vi "XLP80_FGlob_CalculatedAnalog.vi"(5 "Function (Recall One)":T2=enum."Recall one", 7 "CalculatedAnalog_Items":T1, 8 "err in":errorcluster caption="error", 10 "Calc Values IN":sgl[](array[numeric]) format="%.6f", 11 "Calc Value IN":sgl format="%.6f") -> (0 "err out":errorcluster caption="error", 2 "Calc Values OUT":sgl[](array[numeric]) format="%.6f", 3 "Calc Value OUT":sgl format="%.6f")   [LabVIEW 2021]
uses:
  1886_FGlob_TDefs_Enum_FGlobItems.ctl
  XLP80_FGLob_TDefEnumCalcAnalogItems.ctl
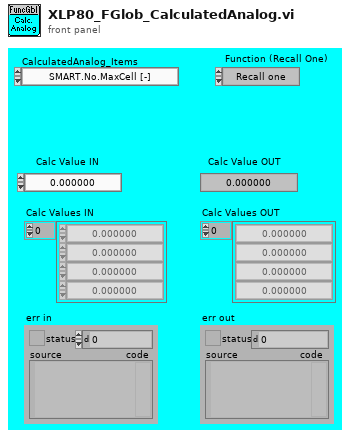
[diagram p1: front panel]
types:
  T1 = typedef "XLP80_FGLob_TDefEnumCalcAnalogItems.ctl" = enum8{"SMART.No.MaxCell [-]", "SMART.No.MinCell [-]", "SMART.U.S.AveCell [V]", "SMART.U.S.CVM [V]", "SMART.U.S.MaxCell [V]", "SMART.U.S.MinCell [V]"}
  T2 = typedef "1886_FGlob_TDefs_Enum_FGlobItems.ctl" = enum16{"Put one", "Put all", "Recall one", "Recall all"}
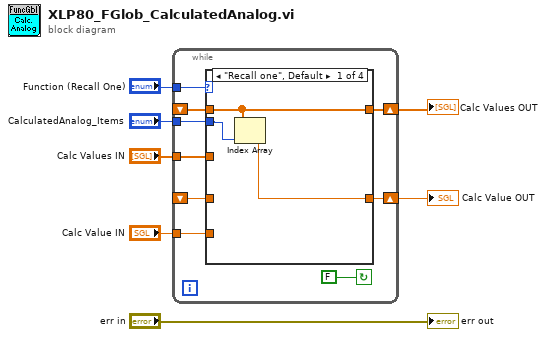
[diagram p0: block diagram]
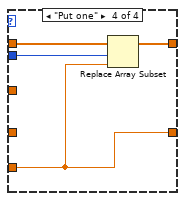
[diagram p4: hidden frame]
diagram:
  n1 = while {
    shift-right: [w14] -> w5
    shift-left: _ -> [w13]
    tunnel: "Function (Recall One)" -> [w15]
    tunnel: "CalculatedAnalog_Items" -> [w11]
    tunnel: "Calc Values IN" -> [w10]
    shift-right: [w12] -> w4
    shift-left: _ -> [w9]
    tunnel: "Calc Value IN" -> [w8]
    stop <- FALSE continue-if-true
    n2 = case shown="\"Recall one\", Default" w15 {
      tunnel: [w19 w21 w23 w26] -> w14
      tunnel: w13 -> [w19 w21 _ w27]
      tunnel: w11 -> [w18 _ _ w25]
      tunnel: [w17 w20 w22 w24] -> w12
      tunnel: w10 -> [_ _ w23 _]
      tunnel: w9 -> [_ w20 w22 _]
      tunnel: w8 -> [_ _ _ w24]
      frame "Recall one", Default {
        n3 = Index Array(array=w19, index=w18) -> (element=w17:sgl)
      }
      frame "Recall all" {
      }
      frame "Put all" {
      }
      frame "Put one" {
        n4 = Replace Array Subset(array=w27, new element=w24, index=w25) -> (w26:sgl[])
      }
    }
  }
  "Calc Values OUT" <- w5
  "Calc Value OUT" <- w4
  "err out" <- "err in"
